vi "Filter String_Focus Handler.vi"(5 "Disable":bool, 6 "Text Colors":T2={"Enabled Color"=0, "Disabled Color"=10395294}, 7 "Make key focus?":bool, 10 "Default Value":string="Filter...", 11 "Filter String Ref":refnum<vi>) -> ()   [LabVIEW 2023]
doc: "Called asynchronously, this VI sets the default string (default=\"Filter...\") and the secondary color to the control's text color (default = gray), then monitors the control for a change in focus. When control gains focus, it removes the default string and sets the text to the main text color. When it loses focus, and if string is empty, it sets the value to the default and sets secondary text color.\n\nMake key focus will place the cursor before the default text and handle removing default text if user types any ascii character"
uses:
  <vilib>/event_ctls.llb/eventvkey.ctl
panel:
  out "VKey":T1
  in  "Debug Filter String":string
  # "Debug control:"
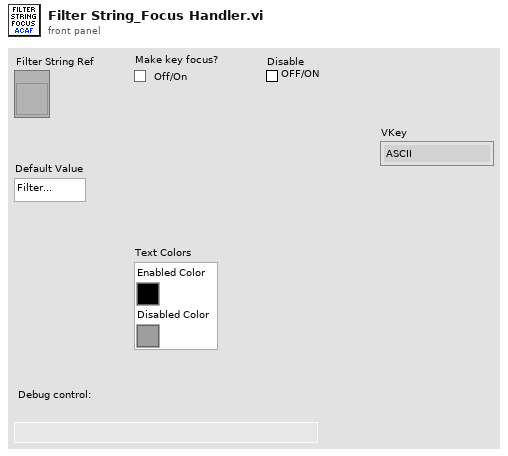
[diagram p1: front panel]
types:
  T1 = typedef "eventvkey.ctl" = enum16{"ASCII", "Enter", "Return", "Shift", "Ctrl", "Alt", "Cmd", "Opt", "Caps", "NumLock", "Clear", "Break", "Up", "Down", "Left", "Right", "Insert", "Delete", "Home", "End", "PageUp", "PageDown", "Escape", "Help", "Pause", "ScrollLock", "F1", "F2", "F3", "F4", "F5", "F6", "F7", "F8", "F9", "F10", "F11", "F12", "F13", "F14", "F15", "F16", "F17", "F18", "F19", "F20", "F21", "F22", "F23", "F24", "Play", "VolumeUp", "VolumeDown", "Mute", "Two Byte Char"}
  T2 = cluster{"Enabled Color":u32, "Disabled Color":u32}
  T3 = enum8{"Enabled", "Disabled", "Disabled and Grayed Out"}
  T4 = cluster{"Selection Start":u32, "Selection End":u32}
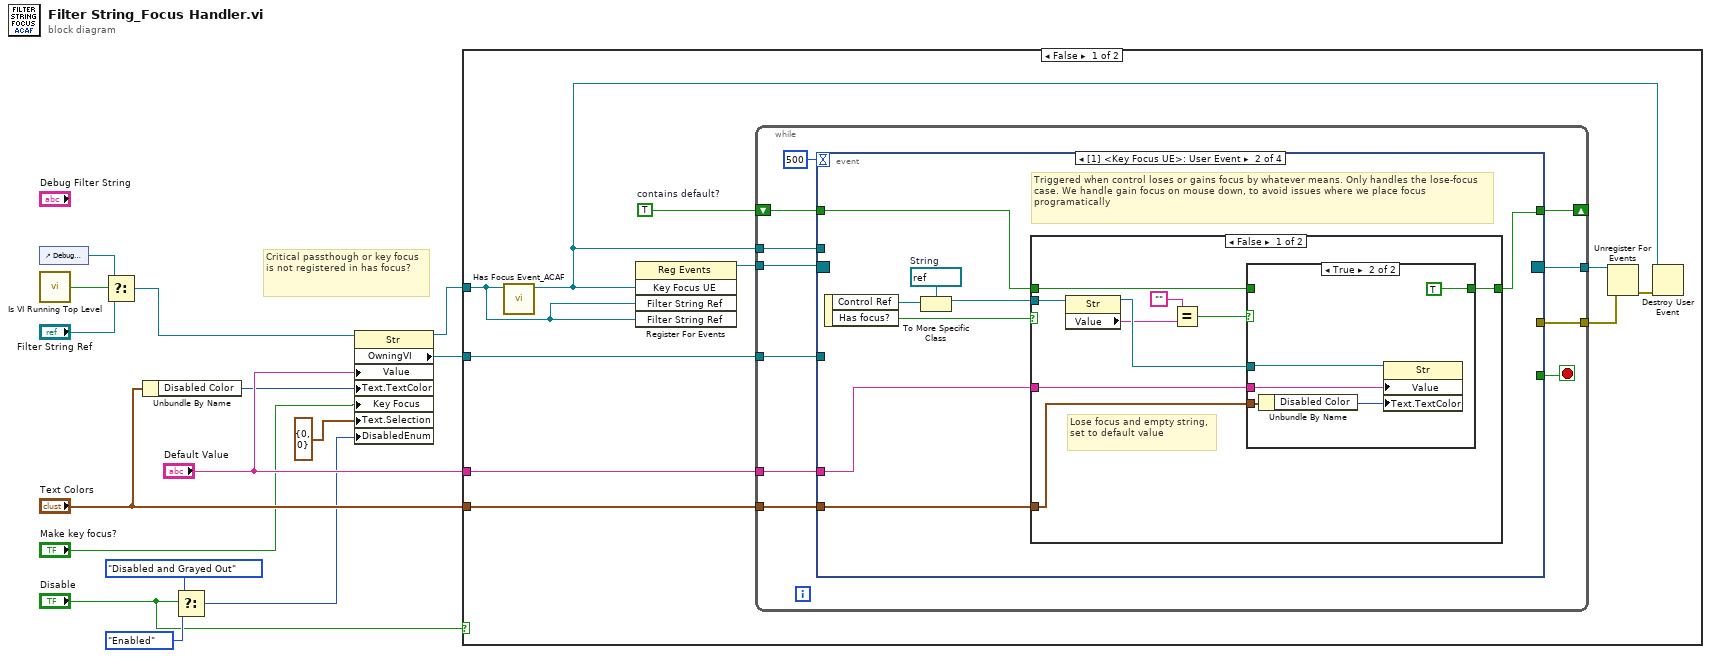
[diagram p0: block diagram]
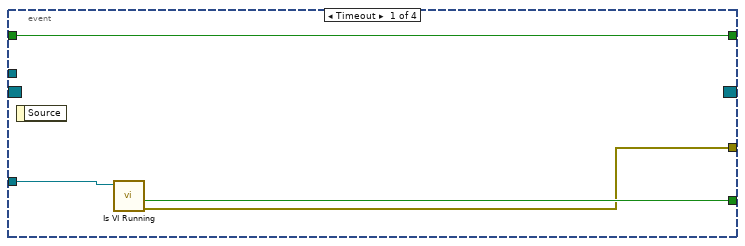
[diagram p2: hidden frame]
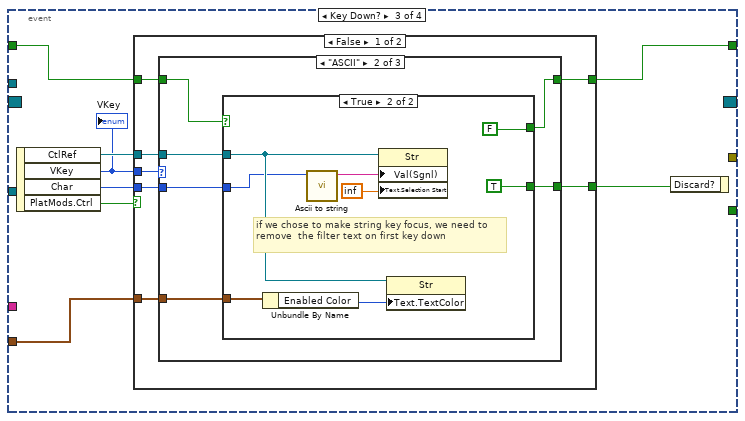
[diagram p5: hidden frame]
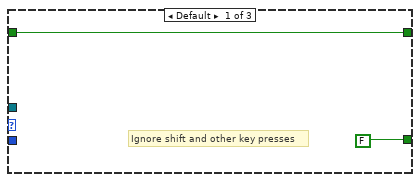
[diagram p6: hidden frame]
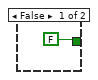
[diagram p7: hidden frame]
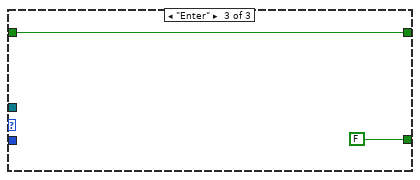
[diagram p8: hidden frame]
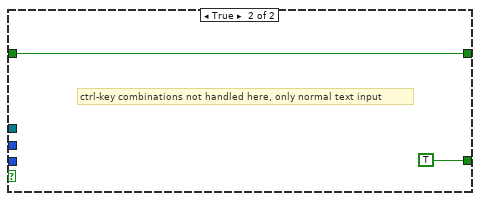
[diagram p9: hidden frame]
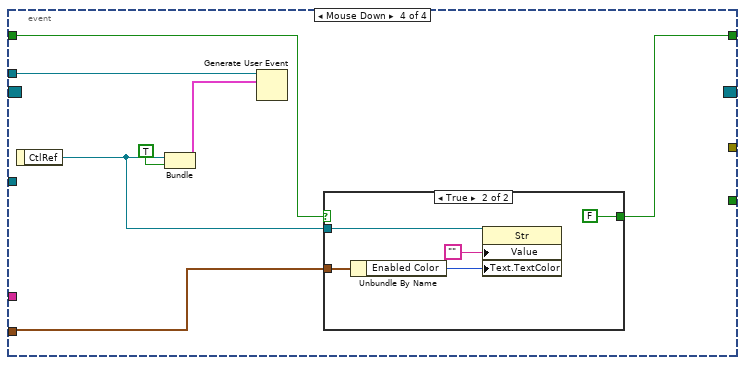
[diagram p10: hidden frame]
diagram:
  # "Critical passthough or key focus is not registered in has focus?"
  n1 = control-ref of="Debug Filter String"() -> (w14:refnum<vi>)
  n2 = call "Is VI Running Top Level.vi"() -> ("Top Level?"=w15:bool)  [unwired: 5 in]
  n3 = Select(t=w14, s=w15, f="Filter String Ref") -> (s? t:f=w2:refnum<vi>)
  n4 = Unbundle By Name("Text Colors") -> ("Disabled Color"=w9:u32)
  n5 = Select(t=T3."Disabled and Grayed Out" ("Disabled"), s="Disable", f=T3."Enabled" ("Disabled")) -> (s? t:f=w4:T3)
  n6 = property class="Str"(reference=w2, "Value"="Default Value", "Text.TextColor"=w9, "Key Focus"="Make key focus?", "Text.Selection"=T4 {"Selection Start"=0, "Selection End"=0}, "DisabledEnum"=w4) -> (reference out=w1:refnum<vi>, "OwningVI"=w11:refnum<vi>)  [unwired: 1 in, 1 out]
  n7 = case shown="False" "Disable" {
    tunnel: "Text Colors" -> [w24 _]
    tunnel: w11 -> [w23 _]
    tunnel: "Default Value" -> [w21 _]
    tunnel: w1 -> [w17 _]
    frame False {
      w22 = TRUE  # contains default?
      n8 = call "Has Focus Event_ACAF.vi"("Control Ref"=w17) -> ("Key Focus UE"=w16:refnum<user-event>)  [unwired: 9 in, 1 out]
      n9 = register-events(w16, w17, w17) -> (reference out=w25:refnum<event-registration>)  [unwired: 2 in, 1 out]
      n10 = while {
        tunnel: w25 -> [w34]
        tunnel: w21 -> [w33]
        tunnel: w24 -> [w32]
        tunnel: w23 -> [w31]
        shift-right: [w29] -> _
        shift-left: w22 -> [w30]
        tunnel: [w28] -> w19
        tunnel: [w27] -> w20
        tunnel: w16 -> [w26]
        stop <- w36 stop-if-true
        n11 = event shown="[1] <Key Focus UE>: User Event" {
          selector: w34 -> [_ _ _ _]
          dyn-events: [_ _ _ _] -> w27
          timeout: 500 -> [_ _ _ _]
          tunnel: [w39 _ _ _] -> w36
          tunnel: w33 -> [_ w47 _ _]
          tunnel: w32 -> [_ w46 w68 w101]
          tunnel: w31 -> [w40 _ _ _]
          tunnel: [w38 w44 w72 w104] -> w29
          tunnel: w30 -> [w38 w45 w71 w103]
          tunnel: [w37 _ _ _] -> w28
          tunnel: w26 -> [_ _ _ w107]
          event Timeout {
            n12 = event-data() -> ()  [unwired: 1 in, 1 out]
            n13 = call "Is VI Running.vi"("VI in"=w40) -> ("error out"=w37:errorcluster, "VI Not Running"=w39:bool)  [unwired: 7 in, 2 out]
          }
          event User Event {
            w42 = refnum<vi> refnum  # String
            # "Triggered when control loses or gains focus by whatever means. Only handles the lose-focus case. We handle gain focus on mouse down, to avoid issues where we place focus programatically"
            n14 = event-data() -> ("Control Ref"=w43:refnum<vi>, "Has focus?"=w48:bool)  [unwired: 1 in]
            n15 = To More Specific Class(target class=w42, reference=w43) -> (specific class reference=w41:refnum<vi>)  [unwired: 1 in, 1 out]
            n16 = case shown="False" w48 {
              tunnel: w47 -> [w54 _]
              tunnel: w46 -> [w53 _]
              tunnel: w45 -> [w49 w64]
              tunnel: [w52 w64] -> w44
              tunnel: w41 -> [w50 _]
              frame False {
                # "Lose focus and empty string, set to default value"
                n17 = property class="Str"(reference=w50) -> (reference out=w56:refnum<vi>, "Value"=w51:string)  [unwired: 1 in, 1 out]
                n18 = Equal?(x="", y=w51) -> (x = y?=w55:bool)
                n19 = case shown="True" w55 {
                  tunnel: w56 -> [_ w59]
                  tunnel: w54 -> [_ w63]
                  tunnel: w53 -> [_ w62]
                  tunnel: [w58 TRUE] -> w52
                  tunnel: w49 -> [w58 _]
                  frame False {
                  }
                  frame True {
                    n20 = Unbundle By Name(w62) -> ("Disabled Color"=w61:u32)
                    n21 = property class="Str"(reference=w59, "Value"=w63, "Text.TextColor"=w61) -> ()  [unwired: 1 in, 2 out]
                  }
                }
              }
              frame True {
              }
            }
          }
          event Key Down? {
            n22 = event-data() -> ("CtlRef"=w70:refnum<vi>, "VKey"=w65:T1, "Char"=w67:i16, "PlatMods.Ctrl"=w66:bool)  [unwired: 1 in]
            "VKey" <- w65
            n23 = case shown="False" w66 {
              tunnel: [w79 w100] -> w72
              tunnel: w71 -> [w78 w100]
              tunnel: w65 -> [w77 _]
              tunnel: w70 -> [w76 _]
              tunnel: [w75 TRUE] -> w69
              tunnel: w68 -> [w74 _]
              tunnel: w67 -> [w73 _]
              frame False {
                n24 = case shown="\"ASCII\"" w77 {
                  tunnel: [w81 w86 w98] -> w79
                  tunnel: w78 -> [w81 w87 w98]
                  tunnel: w76 -> [_ w85 _]
                  tunnel: [FALSE w84 FALSE] -> w75
                  tunnel: w74 -> [_ w83 _]
                  tunnel: w73 -> [_ w82 _]
                  frame Default {
                    # "Ignore shift and other key presses"
                  }
                  frame "ASCII" {
                    n25 = case shown="True" w87 {
                      tunnel: [FALSE FALSE] -> w86
                      tunnel: w85 -> [_ w92]
                      tunnel: [_ TRUE] -> w84
                      tunnel: w83 -> [_ w91]
                      tunnel: w82 -> [_ w89]
                      frame False {
                      }
                      frame True {
                        # "if we chose to make string key focus, we need to remove  the filter text on first key down"
                        n26 = Unbundle By Name(w91) -> ("Enabled Color"=w93:u32)
                        n27 = call "Ascii to string.vi"("ASCII Code"=w89) -> ("String"=w90:string)  [unwired: 10 in]
                        n28 = property class="Str"(reference=w92, "Val(Sgnl)"=w90, "Text.Selection Start"=inf) -> ()  [unwired: 1 in, 2 out]
                        n29 = property class="Str"(reference=w92, "Text.TextColor"=w93) -> ()  [unwired: 1 in, 2 out]
                      }
                    }
                  }
                  frame "Enter" {
                  }
                }
              }
              frame True {
                # "ctrl-key combinations not handled here, only normal text input"
              }
            }
            n30 = event-data("Discard?"=w69) -> ()  [unwired: 1 in, 1 out]
          }
          event Mouse Down {
            n31 = event-data() -> ("CtlRef"=w102:refnum<vi>)  [unwired: 1 in]
            n32 = Bundle("CtlRef"=w102, TRUE) -> (w106:cluster{"CtlRef":refnum<vi>, bool})  [unwired: 1 in]
            n33 = Generate User Event(user event=w107, event data cluster=w106) -> ()  [unwired: 2 in, 2 out]
            n34 = case shown="True" w103 {
              selector: w103 -> [w108 _]
              tunnel: w102 -> [_ w112]
              tunnel: w101 -> [_ w111]
              tunnel: [w108 FALSE] -> w104
              frame False {
              }
              frame True {
                n35 = Unbundle By Name(w111) -> ("Enabled Color"=w110:u32)
                n36 = property class="Str"(reference=w112, "Value"="", "Text.TextColor"=w110) -> ()  [unwired: 1 in, 2 out]
              }
            }
          }
        }
      }
      n37 = Unregister For Events(event registration refnum=w20, error in=w19) -> (error out=w18:errorcluster)
      n38 = Destroy User Event(user event=w16, error in=w18) -> ()  [unwired: 1 out]
    }
    frame True {
    }
  }
